vi "运维调试_总磷总氮.vi"() -> ()   [LabVIEW 2016, in "斯坦道总磷总氮V2.lvlib"]
uses:
  <vilib>/Utility/miscctls.llb/LVPointTypeDef.ctl
  <vilib>/Plasmionique/MB Master/MB_Master/MB_Master.lvclass
  <vilib>/ptbypt/NI_PtbyPt.lvlib
panel:
  in  "流程写入":bool
  in  "修改系列号":bool
  out "权限等级":string
  out "总步数":i32
  out "滑动杆":u8(slide) caption="测试进度" scale=0.0..100.0
  in  "关闭心跳包":bool
  in  "仪器校准":bool
  in  "参数查询":bool
  out "简易步骤名称":string
  in  "温度曲线":bool
  in  "启动参数设置":bool
  out "固件版本号":string
  in  "定时设置":cluster{"启动":bool, "控制命令":T1, "测量参数":T2}(xcontrol)
  out "模块版本号":string
  out "注射器温度":sgl
  out "消解温度":sgl
  out "ADC":sgl
  out "F3":sgl format="%#.6f"
  out "F2":sgl format="%#.6f"
  out "F1":sgl format="%#.6f"
  out "F0":sgl format="%#.6f"
  out "运行状态":T3 {"数据时间:" format="%<%y/%m/%d %H:%M:%S>T"; "仪器时间:" format="%<%y/%m/%d %H:%M:%S>T"}
  in  "单选按钮":T4(radio)=enum."总氮"
  in  "布尔":bool
  out "字符串 2":string
  in  "数组":string[](array[string])
  in  "返回":bool
  in  "参数设置":bool
  out "集成报警信息":string
  in  "停止":bool
  in  "手动启动":bool
  in  "调试":bool
  out "多列列表框":i32(listbox)
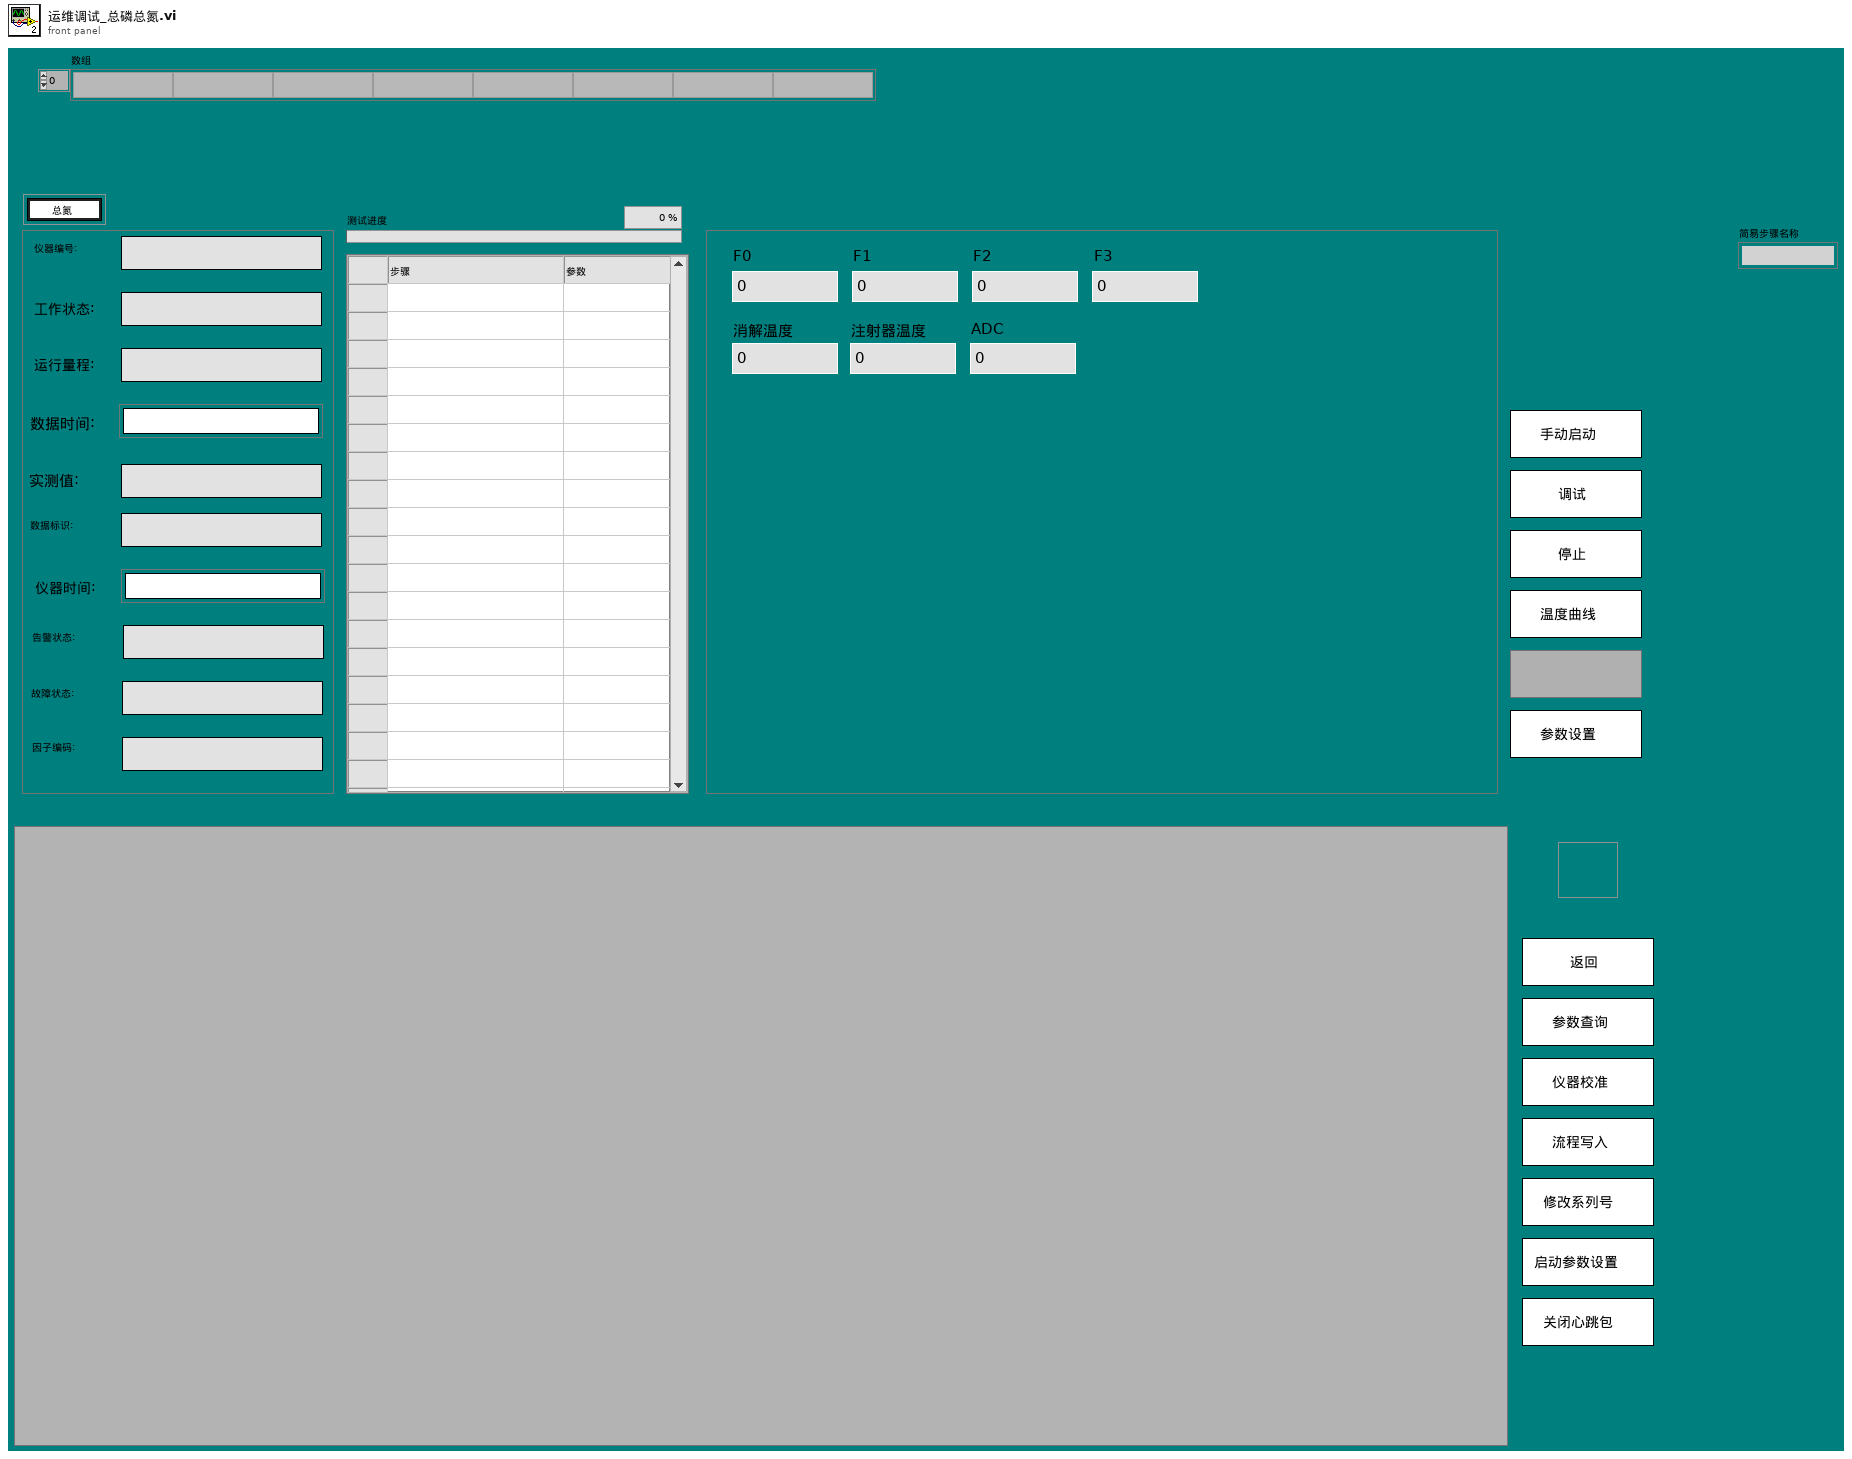
[diagram p1: front panel]
types:
  T1 = typedef "定时设置.xctl/国标控制命令.ctl" = enum16{"启动测量", "标样核查", "零点核查", "跨度核查", "空白测试", "平行样测试", "加标回收", "空白校准", "标样校准", "初始化（清洗）", "停止测试", "仪器重启", "校时", "模式设置", "测量间隔设置"}
  T2 = typedef "定时设置.xctl/测量参数.ctl" = u16
  T3 = cluster{"仪器编号:":string, "工作状态:":string, "运行量程: ":string, "数据时间:":timestamp, "实测值:":string, "数据标识: ":string, "仪器时间:":timestamp, "告警状态: ":string, "故障状态:  ":string, "因子编码:":string}
  T4 = enum32{"COD", "氨氮", "总氮", "总磷", "磷酸盐", "硝氮", "亚硝氮", "硅酸盐", "硫化物"}
  T5 = cluster{"Major":u16, "Minor":u16, "Fix":u16, "Build":u16}
  T6 = typedef "LVPointTypeDef.ctl" = cluster{"Horizontal":i16, "Vertical":i16}
  T7 = cluster{"系统时间":timestamp, "工作状态":u16, "测量模式":enum16{"待机", "连续模式", "周期模式", "定点模式", "受控模式", "手动模式"}, "告警代码":u16, "故障代码":u16, "日志代码":u16, "软件版本":u16, "F0":sgl, "F1":sgl, "F2":sgl, "F3":sgl, "T":sgl, "H":sgl, "id":u16, "flowid":u16, "量程":u16, "总磷控温温度1":sgl, "营养盐控温温度2":sgl, "ADC":sgl}
  T8 = cluster{"因子编码":u32, "单位":u16, "标样参考值":sgl, "水样数据时间":timestamp, "水样实测值":sgl, "水样数据标识":string, "标样数据时间":timestamp, "标样实测值":sgl, "标样数据标识":string, "空白数据时间":timestamp, "空白实测值":sgl, "空白数据标识":string, "零点核查数据时间":timestamp, "零点核查实测值":sgl, "零点核查数据标识":string, "跨度核查数据时间":timestamp, "跨度核查实测值":sgl, "跨度核查数据标识":string, "加标回收数据时间":timestamp, "加标回收实测值":sgl, "加标回收数据标识":string, "平行样数据时间":timestamp, "平行样实测值":sgl, "平行样数据标识":string, "F0":sgl, "F1":sgl, "F2":sgl, "F3":sgl, "F4":sgl, "F5":sgl, "F6":sgl, "F7":sgl, "温度":sgl, "湿度":sgl, "X值":sgl, "fidrange":u16}[]
  T9 = cluster{"因子编码":u32, "单位":u16, "标样参考值":sgl, "水样数据时间":timestamp, "水样实测值":sgl, "水样数据标识":string, "标样数据时间":timestamp, "标样实测值":sgl, "标样数据标识":string, "空白数据时间":timestamp, "空白实测值":sgl, "空白数据标识":string, "零点核查数据时间":timestamp, "零点核查实测值":sgl, "零点核查数据标识":string, "跨度核查数据时间":timestamp, "跨度核查实测值":sgl, "跨度核查数据标识":string, "加标回收数据时间":timestamp, "加标回收实测值":sgl, "加标回收数据标识":string, "平行样数据时间":timestamp, "平行样实测值":sgl, "平行样数据标识":string, "F0":sgl, "F1":sgl, "F2":sgl, "F3":sgl, "F4":sgl, "F5":sgl, "F6":sgl, "F7":sgl, "温度":sgl, "湿度":sgl, "X值":sgl, "fidrange":u16}
  T10 = cluster{"时间标识":timestamp, "设备":string, "日志信息":string, "备注":string}
  T11 = cluster{"参数":string, "报警内容":string, "报警分析":string}
  T12 = enum32{"Bad", "Idle", "Run top level", "Running"}
  T13 = enum16{"空闲", "水样测试", "标样核查", "零点核查", "跨度核查", "空白测试", "平行样测试", "加标回收", "空白校准", "标样校准", "初始化（清洗）"}
  T14 = cluster{"站号":u16, "量程切换":enum32{"H", "L", "AUTO"}, "控制命令":enum16{"启动测量", "标样核查", "零点核查", "跨度核查", "空白测试", "平行样测试", "加标回收", "空白校准", "标样校准", "初始化（清洗）", "停止测试", "仪器重启", "校时", "模式设置", "测量间隔设置"}, "模式设置":enum16{"待机", "连续模式", "周期模式", "定点模式", "受控模式", "手动模式"}, "测量间隔":u16}
  T15 = cluster{"时间标识":timestamp, "设备":string, "日志信息":string, "流程参数":string}
  T16 = typedef "LVRowAndColumnUnsignedTypeDef.ctl" = cluster{"Row":u32, "Column":u32}
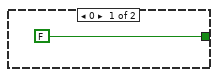
[diagram p3: hidden frame]
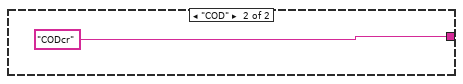
[diagram p4: hidden frame]
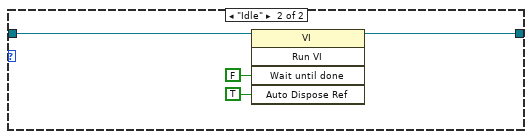
[diagram p7: hidden frame]
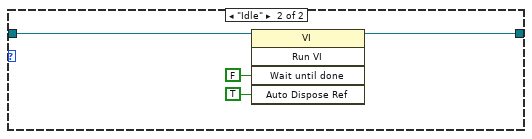
[diagram p8: hidden frame]
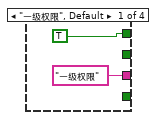
[diagram p14: hidden frame]
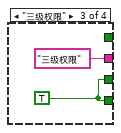
[diagram p15: hidden frame]
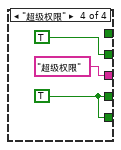
[diagram p16: hidden frame]
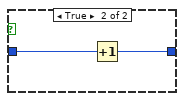
[diagram p18: hidden frame]
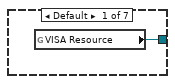
[diagram p20: hidden frame]
diagram:
  n1 = flat-sequence {
    tunnel: [w28] -> w17
    tunnel: [w29] -> w16
    tunnel: w17 -> [w40]
    tunnel: [w40] -> w2
    tunnel: w16 -> [_]
    tunnel: w2 -> [w63]
    tunnel: [w111] -> w18
    tunnel: [errorcluster {"status"=FALSE, "code"=0, "source"=""} ("错误输入（无错误）")] -> w7
    tunnel: [errorcluster {"status"=FALSE, "code"=0, "source"=""} ("错误输入（无错误）")] -> w6
    tunnel: [w108] -> w4
    tunnel: [errorcluster {"status"=FALSE, "code"=0, "source"=""} ("error out")] -> w1
    tunnel: [errorcluster {"status"=FALSE, "code"=0, "source"=""} ("错误输入（无错误）")] -> w3
    frame #0 {
      n2 = control-ref of="本VI"() -> (w30:refnum<vi>)
      n3 = control-ref of="本VI"() -> (w39:refnum<vi>)
      n4 = call "配置读取.vi"() -> ("error out"=w29:errorcluster)  [unwired: 11 in]
      n5 = property class="VI"(reference=w30) -> ("Library"=w31:refnum<vi>)  [unwired: 1 in, 2 out]
      n6 = property class="VI"(reference=w39) -> ("Library.Version"=w38:T5)  [unwired: 1 in, 2 out]
      n7 = property class="Library"(reference=w31) -> ("LocalName"=w28:string)  [unwired: 1 in, 2 out]
      n8 = Unbundle By Name(w38) -> ("Major"=w36:u16, "Minor"=w35:u16, "Fix"=w34:u16, "Build"=w33:u16)
      n9 = Search/Split String(string=w28, search string/char (-)="." ("搜索字符串/字符(-)")) -> (substring before match=w26:string)  [unwired: 1 in, 2 out]
      n10 = property on="定时设置" class="定时设置 (严格)"("调用模块名称写入"=w26) -> ()  [unwired: 2 in, 2 out]
      n11 = Format Into String(format string="模块版本号：%d.%d.%d.%d" ("格式字符串"), w36, w35, w34, w33) -> (resulting string=→"模块版本号":string)  [unwired: 2 in, 1 out]
    }
    frame #1 {
      n12 = global read "总磷总氮断电保存全局变量.vi" "IP"() -> (w44:string)
      n13 = global read "总磷总氮断电保存全局变量.vi" "VISA Resource"() -> (w41:refnum<visa-resource-name>)
      n14 = Empty String/Path?(string/path=w44) -> (empty?=w43:bool)
      n15 = Empty String/Path?(string/path=w41) -> (empty?=w42:bool)
      n16 = case shown="真" w43 {
        tunnel: w40 -> [_ w55]
        frame False {
        }
        frame True {
          n17 = case shown="\"斯坦道CODcrV2.lvlib\"" w55 {
            tunnel: [w56 "192.168.1.203" ("IP") "192.168.1.202" ("IP") "192.168.1.202" ("IP") "192.168.1.203" ("IP") "192.168.1.204" ("IP") "192.168.1.205" ("IP")] -> w54
            frame Default {
              n18 = global read "总磷总氮断电保存全局变量.vi" "IP"() -> (w56:string)
            }
            frame "斯坦道总磷总氮V2.lvlib" {
            }
            frame "斯坦道氨氮V2.lvlib" {
            }
            frame "斯坦道氨氮总磷V2.lvlib" {
            }
            frame "斯坦道总磷V2.lvlib" {
            }
            frame "斯坦道总氮V2.lvlib" {
            }
            frame "斯坦道CODcrV2.lvlib" {
            }
          }
          n19 = global write "总磷总氮断电保存全局变量.vi" "IP"(w54) -> ()
        }
      }
      n20 = case shown="真" w42 {
        tunnel: w40 -> [_ w46]
        frame False {
        }
        frame True {
          n21 = case shown="\"斯坦道总磷V2.lvlib\"" w46 {
            tunnel: [w47 "COM5" ("IP") "COM7" ("IP") "COM7" ("IP") "COM5" ("IP") "COM10" ("IP") "COM9" ("IP")] -> w45
            frame Default {
              n22 = global read "总磷总氮断电保存全局变量.vi" "VISA Resource"() -> (w47:refnum<visa-resource-name>)
            }
            frame "斯坦道总磷总氮V2.lvlib" {
            }
            frame "斯坦道氨氮V2.lvlib" {
            }
            frame "斯坦道氨氮总磷V2.lvlib" {
            }
            frame "斯坦道总磷V2.lvlib" {
            }
            frame "斯坦道总氮V2.lvlib" {
            }
            frame "斯坦道CODcrV2.lvlib" {
            }
          }
          n23 = global write "总磷总氮断电保存全局变量.vi" "VISA Resource"(w45) -> ()
        }
      }
    }
    frame #2 {
      n24 = global read "总磷总氮断电保存全局变量.vi" "启动队列名称"() -> (w65:cluster{"String":string, "Value":u16}[])
      n25 = Empty Array?(array=w65) -> (empty?=w64:bool)
      n26 = case shown="真" w64 {
        tunnel: w63 -> [_ w66]
        frame False {
        }
        frame True {
          n27 = case shown="\"斯坦道总氮V2.lvlib\"" w66 {
            frame Default {
            }
            frame "斯坦道总磷总氮V2.lvlib" {
              n28 = global write "总磷总氮断电保存全局变量.vi" "启动队列名称"(cluster{"String":string, "Value":u16}[] [{"String"="总氮", "Value"=2}, {"String"="总磷", "Value"=1}] ("启动队列名称")) -> ()
            }
            frame "斯坦道氨氮V2.lvlib" {
              n29 = global write "总磷总氮断电保存全局变量.vi" "启动队列名称"(cluster{"String":string, "Value":u16}[] [{"String"="氨氮", "Value"=3}] ("启动队列名称")) -> ()
            }
            frame "斯坦道氨氮总磷V2.lvlib" {
              n30 = global write "总磷总氮断电保存全局变量.vi" "启动队列名称"(cluster{"String":string, "Value":u16}[] [{"String"="氨氮", "Value"=3}, {"String"="总磷", "Value"=1}] ("启动队列名称")) -> ()
            }
            frame "斯坦道总磷V2.lvlib" {
              n31 = global write "总磷总氮断电保存全局变量.vi" "启动队列名称"(cluster{"String":string, "Value":u16}[] [{"String"="总磷", "Value"=1}] ("启动队列名称")) -> ()
            }
            frame "斯坦道总氮V2.lvlib" {
              n32 = global write "总磷总氮断电保存全局变量.vi" "启动队列名称"(cluster{"String":string, "Value":u16}[] [{"String"="总氮", "Value"=2}] ("启动队列名称")) -> ()
            }
            frame "斯坦道CODcrV2.lvlib" {
              n33 = global write "总磷总氮断电保存全局变量.vi" "启动队列名称"(cluster{"String":string, "Value":u16}[] [{"String"="CODcr", "Value"=22}] ("启动队列名称")) -> ()
            }
          }
        }
      }
    }
    frame #3 {
      # "初始化"
      n34 = global read "总磷总氮断电保存全局变量.vi" "流程路径"() -> (w76:path)
      n35 = global read "总磷总氮断电保存全局变量.vi" "启动队列名称"() -> (w73:cluster{"String":string, "Value":u16}[])
      n36 = call <vilib>:"Check if File or Folder Exists.vi"("path"=w76) -> ("file or folder exists?"=w80:bool)  [unwired: 8 in, 2 out]
      n37 = for {
        tunnel: w73 -> [w84] mode=indexing
        shift-right: [w83] -> w74
        shift-left: "" -> [w81]
        n38 = Unbundle By Name(w84) -> ("String"=w82:string)
        n39 = Concatenate Strings(w81, w82) -> (w83:string)
      }
      n40 = Empty String/Path?(string/path=w76) -> (empty?=w77:bool)
      n41 = Not(x=w80) -> (.not. x?=w79:bool)
      n42 = Or(x=w77, y=w79) -> (x .or. y?=w78:bool)
      n43 = case shown="真" w78 {
        frame False {
        }
        frame True {
          n44 = global read "总磷总氮断电保存全局变量.vi" "启动队列名称"() -> (w86:cluster{"String":string, "Value":u16}[])
          n45 = for {
            tunnel: w86 -> [w89] mode=indexing
            tunnel: [w88] -> w85 mode=indexing
            n46 = Unbundle By Name(w89) -> ("String"=w88:string)
          }
          n47 = call "获取默认流程路径.vi"("参数"=w85) -> ("路径"=w87:path)  [unwired: 10 in]
          n48 = global write "总磷总氮断电保存全局变量.vi" "流程路径"(w87) -> ()
        }
      }
      n49 = global write "VAR总磷总氮全局变量.vi" "模块名称"(w74) -> ()
    }
    frame #4 {
      n50 = vi-ref "总磷总氮测量数据储存.vi"() -> (w98:refnum<vi>)
      n51 = vi-ref "总磷总氮通讯.vi"() -> (w90:refnum<vi>)
      n52 = property class="VI"(reference=w98) -> ("Name"=w105:string)  [unwired: 1 in, 2 out]
      n53 = property class="VI"(reference=w90) -> ("Name"=w91:string)  [unwired: 1 in, 2 out]
      n54 = Open VI Reference(type specifier VI Refnum (for type only)=refnum<vi> refnum, vi path=w105, options=128 ("选项")) -> (vi reference=w103:refnum<vi>, error out=w101:errorcluster)  [unwired: 3 in]
      n55 = Open VI Reference(type specifier VI Refnum (for type only)=refnum<vi> refnum, vi path=w91, options=128 ("选项")) -> (vi reference=w93:refnum<vi>, error out=w95:errorcluster)  [unwired: 3 in]
      n56 = call-by-ref "开始异步调用"(reference=w103, error in=w101) -> (reference out=w99:refnum<vi>, error out=w100:errorcluster)  [unwired: 12 in]
      n57 = call-by-ref "开始异步调用"(reference=w93, error in=w95) -> (reference out=w97:refnum<vi>, error out=w96:errorcluster)  [unwired: 12 in]
      n58 = Close Reference(reference=w99, error in (no error)=w100) -> ()  [unwired: 1 out]
      n59 = Close Reference(reference=w97, error in (no error)=w96) -> ()  [unwired: 1 out]
    }
    frame #5 {
      n60 = call "配置文件路径.vi"() -> ("appended path"=w108:path)  [unwired: 11 in]
      n61 = call "设置模块队列名.vi"() -> ("Msg"=w111:string)  [unwired: 5 in]
    }
  }
  n62 = flat-sequence {
    frame #0 {
      n63 = property on="窗格" class="Pane"("Origin"=T6 {"Horizontal"=0, "Vertical"=0} ("原点")) -> ()  [unwired: 2 in, 2 out]
    }
  }
  n64 = while {
    shift-right: [w116] -> _
    shift-left: _ -> [w114]
    stop <- FALSE stop-if-true
    n65 = global read "VAR总磷总氮全局变量.vi" "状态告警区"() -> (w138:T7)
    n66 = global read "VAR总磷总氮全局变量.vi" "通讯状态"() -> (w149:bool)
    n67 = global write "VAR总磷总氮全局变量.vi" "最近一次工作状态"(w114) -> ()
    n68 = global read "VAR总磷总氮全局变量.vi" "状态告警区"() -> (w147:T7)
    n69 = Unbundle By Name(w138) -> ("id"=w137:u16, "工作状态"=w132:u16)
    n70 = case shown="真" w149 {
      tunnel: ["通讯异常" ("集成报警信息") w243] -> w148
      frame False {
      }
      frame True {
        n71 = global read "VAR总磷总氮全局变量.vi" "状态告警区"() -> (w249:T7)
        n72 = Unbundle By Name(w249) -> ("工作状态"=w248:u16)
        n73 = feedback #1(0) -> (w246:i32)
        n74 = case shown="0" w248 {
          tunnel: w246 -> [_ w251]
          tunnel: [_ w250] -> w244
          frame 0 {
          }
          frame Default {
            n75 = Increment(x=w251) -> (x+1=w250:i32)
          }
        }
        n76 = feedback-in #1(w244) -> ()
        n77 = global read "VAR总磷总氮全局变量.vi" "测量状态"() -> (w242:string)
        n78 = Format Into String(format string="工作计时: %d 秒" ("格式字符串"), initial string=w242, w244) -> (resulting string=w243:string)  [unwired: 1 in, 1 out]
      }
    }
    "集成报警信息" <- w148
    n79 = Unbundle By Name(w147) -> ("flowid"=w113:u16, "系统时间"=w143:timestamp, "工作状态"=w142:u16, "告警代码"=w136:u16, "故障代码"=w134:u16, "量程"=w141:u16)
    n80 = case shown="\"氨氮\"" "单选按钮" {
      tunnel: [22 3 2 1 4 5 6 7 8] -> w117
      frame "COD", Default {
      }
      frame "氨氮" {
      }
      frame "总氮" {
      }
      frame "总磷" {
      }
      frame "磷酸盐" {
      }
      frame "硝氮" {
      }
      frame "亚硝氮" {
      }
      frame "硅酸盐" {
      }
      frame "硫化物" {
      }
    }
    n81 = case shown="1, 默认" w132 {
      tunnel: w137 -> [_ w194]
      frame 0 {
      }
      frame 1, Default {
        n82 = case shown="3, 92" w194 {
          frame 0, Default {
          }
          frame 1, 131 {
            n83 = local write "单选按钮"(T4."总磷" ("单选按钮")) -> ()
          }
          frame 2, 76 {
            n84 = local write "单选按钮"(T4."总氮" ("单选按钮")) -> ()
          }
          frame 22 {
            n85 = local write "单选按钮"(T4."COD" ("单选按钮")) -> ()
          }
          frame 3, 92 {
            n86 = local write "单选按钮"(T4."氨氮" ("单选按钮")) -> ()
          }
          frame 4 {
            n87 = local write "单选按钮"(T4."磷酸盐" ("单选按钮")) -> ()
          }
          frame 5 {
            n88 = local write "单选按钮"(T4."硝氮" ("单选按钮")) -> ()
          }
          frame 6 {
            n89 = local write "单选按钮"(T4."亚硝氮" ("单选按钮")) -> ()
          }
          frame 7 {
            n90 = local write "单选按钮"(T4."硅酸盐" ("单选按钮")) -> ()
          }
          frame 8 {
            n91 = local write "单选按钮"(T4."硫化物" ("单选按钮")) -> ()
          }
        }
      }
    }
    n92 = case shown="255" w142 {
      selector: w142 -> [w208 _ w214 w218 w221 w223 w225 w227 w229 w231 w233 w235 w237 w240]
      tunnel: [w209 "空闲" ("工作状态") "水样测量" ("工作状态") w217 "零点核查" ("工作状态") "跨度核查" ("工作状态") "空白测试" ("工作状态") "平行样测试" ("工作状态") "加标回收" ("工作状态") "空白校准" ("工作状态") "标样校准" ("工作状态") "初始化" ("工作状态") "单步调试" ("工作状态") w239] -> w115
      tunnel: [w207 w212 w214 w218 w221 w223 w225 w227 w229 w231 w233 w235 w237 w240] -> w116
      tunnel: w114 -> [w207 w212 _ _ _ _ _ _ _ _ _ _ _ _]
      tunnel: w113 -> [_ _ _ w216 _ _ _ _ _ _ _ _ _ _]
      frame Default {
        n93 = Format Into String(format string="%d" ("格式字符串"), initial string="未知" ("工作状态"), w208) -> (resulting string=w209:string)  [unwired: 1 in, 1 out]
      }
      frame 0 {
      }
      frame 1 {
      }
      frame 2 {
        n94 = case shown="5" w216 {
          tunnel: ["标样核查" ("工作状态") "快捷测试" ("工作状态")] -> w217
          frame 0, Default {
          }
          frame 5 {
          }
        }
      }
      frame 3 {
      }
      frame 4 {
      }
      frame 5 {
      }
      frame 6 {
      }
      frame 7 {
      }
      frame 8 {
      }
      frame 9 {
      }
      frame 10 {
      }
      frame 254 {
      }
      frame 255 {
        n95 = local read "简易步骤名称"() -> (w239:string)
      }
    }
    n96 = case shown="1" w141 {
      tunnel: ["" ("字符串") "低量程 " ("字符串") "高量程 " ("字符串")] -> w140
      frame Default {
      }
      frame 0 {
      }
      frame 1 {
      }
    }
    n97 = Wait (ms)(milliseconds to wait=u32 1000 ("等待时间（毫秒）")) -> ()  [unwired: 1 out]
    n98 = call "id参数转换.vi"("id"=w117) -> ("数组资源索引"=w118:i32)  [unwired: 9 in, 1 out]
    n99 = global read "VAR总磷总氮全局变量.vi" "测量数据区数组"() -> (w121:T8)
    n100 = Index Array(array=w121, index=w118) -> (element=w120:T9)
    n101 = case shown="0, 默认" w114 {
      tunnel: [w163 w169 w173 w177 w181 w185 w189 w193] -> w131
      tunnel: [w161 w168 w172 w176 w179 w184 w188 w192] -> w126
      tunnel: [w164 w167 w171 w175 w178 w183 w187 w191] -> w124
      tunnel: w120 -> [_ w166 w170 w174 w180 w182 w186 w190]
      frame 0, Default {
        n102 = local read "运行状态"() -> (w165:T3)
        n103 = Unbundle By Name(w165) -> ("数据时间:"=w163:timestamp, "实测值:"=w162:string, "数据标识:"=w164:string)
        n104 = Fract/Exp String To Number(string=w162) -> (number=w161:dbl)  [unwired: 3 in, 1 out]
      }
      frame 1 {
        n105 = Unbundle By Name(w166) -> ("水样数据时间"=w169:timestamp, "水样实测值"=w168:sgl, "水样数据标识"=w167:string)
      }
      frame 2, 9 {
        n106 = Unbundle By Name(w170) -> ("标样数据时间"=w173:timestamp, "标样实测值"=w172:sgl, "标样数据标识"=w171:string)
      }
      frame 3 {
        n107 = Unbundle By Name(w174) -> ("零点核查数据时间"=w177:timestamp, "零点核查实测值"=w176:sgl, "零点核查数据标识"=w175:string)
      }
      frame 4 {
        n108 = Unbundle By Name(w180) -> ("跨度核查数据时间"=w181:timestamp, "跨度核查实测值"=w179:sgl, "跨度核查数据标识"=w178:string)
      }
      frame 7 {
        n109 = Unbundle By Name(w182) -> ("加标回收数据时间"=w185:timestamp, "加标回收实测值"=w184:sgl, "加标回收数据标识"=w183:string)
      }
      frame 5, 8 {
        n110 = Unbundle By Name(w186) -> ("空白数据时间"=w189:timestamp, "空白实测值"=w188:sgl, "空白数据标识"=w187:string)
      }
      frame 6 {
        n111 = Unbundle By Name(w190) -> ("平行样数据时间"=w193:timestamp, "平行样实测值"=w192:sgl, "平行样数据标识"=w191:string)
      }
    }
    n112 = Unbundle By Name(w120) -> ("因子编码"=w122:u32)
    n113 = global write "VAR总磷总氮全局变量.vi" "工作状态:"(w115) -> ()
    n114 = Format Into String(format string="w%05d" ("格式字符串"), w122) -> (resulting string=w139:string)  [unwired: 2 in, 1 out]
    n115 = Number To Fractional String(number=w126, precision (6)=i16 4 ("精度(6)")) -> (F-format string=w128:string)  [unwired: 2 in]
    n116 = call "告警码字段定义.vi"("告警代码"=w136) -> ("字符串"=w135:string)  [unwired: 8 in, 2 out]
    n117 = call "故障码字段定义.vi"("故障代码"=w134) -> ("字符串"=w133:string)  [unwired: 10 in]
    n118 = Concatenate Strings(w128, " " ("字符串"), "mg/L" ("字符串")) -> (w125:string)
    n119 = global read "VAR总磷总氮全局变量.vi" "序列号"() -> (w144:string)
    n120 = Bundle By Name(cluster=T3 {"仪器编号:"="", "工作状态:"="", "运行量程: "="", "数据时间:"=timestamp(0 s since 1904-01-01), "实测值:"="", "数据标识: "="", "仪器时间:"=timestamp(0 s since 1904-01-01), "告警状态: "="", "故障状态:  "="", "因子编码:"=""} ("运行状态"), "仪器编号:"=w144, "仪器时间:"=w143, "工作状态:"=w115, "告警状态:"=w135, "故障状态:"=w133, "运行量程:"=w140, "数据时间:"=w131, "实测值:"=w125, "数据标识:"=w124, "因子编码:"=w139) -> (→"运行状态":T3)
  }
  n121 = call "Create balloon 队列.vi"() -> ("队列输出"=w22:refnum<queue>)  [unwired: 11 in]
  n122 = while {
    shift-right: [w255] -> _
    shift-left: _ -> [w254]
    stop <- FALSE stop-if-true
    n123 = global read "VAR总磷总氮全局变量.vi" "状态告警区"() -> (w257:T7)
    n124 = Unbundle By Name(w257) -> ("工作状态"=w256:u16, "总磷控温温度1"=w253:sgl, "营养盐控温温度2"=w252:sgl)
    n125 = case shown="默认" w256 {
      tunnel: [TRUE _] -> w255
      tunnel: w254 -> [w266 _]
      tunnel: w253 -> [w264 _]
      tunnel: w252 -> [w262 _]
      frame Default {
        n126 = case shown="真" w266 {
          tunnel: [_ w269] -> w265
          tunnel: [_ w268] -> w263
          frame False {
          }
          frame True {
            n127 = global read "VAR总磷总氮全局变量.vi" "波形图-消解温度"() -> (w269:dbl[])
            n128 = global read "VAR总磷总氮全局变量.vi" "波形图-注射器温度"() -> (w268:dbl[])
          }
        }
        n129 = Insert Into Array(array=w265, new element=w264) -> (w261:dbl[])  [unwired: 1 in]
        n130 = Insert Into Array(array=w263, new element=w262) -> (w260:dbl[])  [unwired: 1 in]
        n131 = global write "VAR总磷总氮全局变量.vi" "波形图-消解温度"(w261) -> ()
        n132 = global write "VAR总磷总氮全局变量.vi" "波形图-注射器温度"(w260) -> ()
      }
      frame 0, 254, 255 {
      }
    }
    n133 = Wait (ms)(milliseconds to wait=u32 1000 ("等待时间（毫秒）")) -> ()  [unwired: 1 out]
  }
  n134 = while {
    shift-right: [w280] -> _
    shift-left: u32 0 ("y") -> [w282]
    stop <- FALSE stop-if-true
    # "密码权限"
    n135 = global read "VAR总磷总氮全局变量.vi" "权限等级"() -> (w277:enum16{"一级权限", "二级权限", "三级权限", "超级权限"})
    n136 = case shown="\"二级权限\"" w277 {
      tunnel: [_ TRUE w289 w292] -> w270
      tunnel: [_ _ w289 w292] -> w271
      tunnel: [_ _ _ TRUE] -> w276
      tunnel: [TRUE _ _ _] -> w274
      tunnel: ["一级权限" "二级权限" "三级权限" "超级权限"] -> w272
      frame "一级权限", Default {
      }
      frame "二级权限" {
      }
      frame "三级权限" {
        w289 = TRUE
      }
      frame "超级权限" {
        w292 = TRUE
      }
    }
    "权限等级" <- w272
    n137 = case shown="假" "布尔" {
      tunnel: w282 -> [_ w295]
      tunnel: [_ w294] -> w280
      frame False {
      }
      frame True {
        n138 = Increment(x=w295) -> (x+1=w294:u32)
      }
    }
    n139 = Wait (ms)(milliseconds to wait=u32 1000 ("等待时间（毫秒）")) -> ()  [unwired: 1 out]
    n140 = Not(x=w274) -> (.not. x?=w273:bool)
    n141 = property on="关闭心跳包" class="Bool (严格)"("Visible"=w276) -> ()  [unwired: 2 in, 2 out]
    n142 = property on="流程写入" class="Bool"("Visible"=w270) -> ()  [unwired: 2 in, 2 out]
    n143 = property on="修改系列号" class="Bool"("Visible"=w271) -> ()  [unwired: 2 in, 2 out]
    n144 = property on="启动参数设置" class="Bool"("Visible"=w271) -> ()  [unwired: 2 in, 2 out]
    n145 = Greater Or Equal?(x=w280, y=u32 3600) -> (x >= y?=w278:bool)
    n146 = property on="布尔" class="Bool (严格)"("Value"=w273) -> ()  [unwired: 2 in, 2 out]
    n147 = case shown="真" w278 {
      frame False {
      }
      frame True {
        n148 = global write "VAR总磷总氮全局变量.vi" "权限等级"(enum16{"一级权限", "二级权限", "三级权限", "超级权限"}."一级权限" ("权限等级")) -> ()
      }
    }
  }
  n149 = while {
    shift-right: [w300] -> _
    shift-left: 0 -> [w301]
    stop <- FALSE stop-if-true
    n150 = global read "VAR总磷总氮全局变量.vi" "心跳包打开状态"() -> (w296:bool)
    n151 = case shown="假" w296 {
      tunnel: w301 -> [w305 _]
      tunnel: [w304 _] -> w300
      frame False {
        n152 = Increment(x=w305) -> (x+1=w304:i32)
      }
      frame True {
      }
    }
    n153 = Wait (ms)(milliseconds to wait=u32 1000 ("等待时间（毫秒）")) -> ()  [unwired: 1 out]
    n154 = Greater Or Equal?(x=w300, y=3600) -> (x >= y?=w298:bool)
    n155 = case shown="真" w298 {
      frame False {
      }
      frame True {
        w303 = FALSE ("关闭心跳包")
        n156 = local write "关闭心跳包"(w303) -> ()
        n157 = global write "VAR总磷总氮全局变量.vi" "升级固件关闭心跳包"(w303) -> ()
      }
    }
  }
  n158 = while {
    tunnel: w22 -> [w312]
    shift-right: [w308] -> _
    shift-left: _ -> [w309]
    stop <- FALSE stop-if-true
    n159 = global read "VAR总磷总氮全局变量.vi" "状态告警区"() -> (w306:T7)
    n160 = Unbundle By Name(w306) -> ("工作状态"=w307:u16, "id"=w314:u16, "日志代码"=w313:u16, "故障代码"=w311:u16, "告警代码"=w310:u16)
    n161 = case shown="1, 默认" w307 {
      tunnel: w314 -> [_ w329]
      tunnel: w313 -> [_ w328]
      tunnel: w312 -> [_ w325]
      tunnel: w311 -> [_ w324]
      tunnel: w310 -> [_ w323]
      tunnel: w309 -> [w317 w322]
      tunnel: [w317 w321] -> w308
      frame 0 {
      }
      frame 1, Default {
        n162 = Add(x=w324, y=w323) -> (x+y=w321:u16)
        n163 = call "id参数转换.vi"("id"=w329) -> ("table输出"=w326:string)  [unwired: 9 in, 1 out]
        n164 = Not Equal To 0?(x=w321) -> (x != 0?=w320:bool)
        n165 = Not Equal?(x=w321, y=w322) -> (x != y?=w319:bool)
        n166 = call "故障告警分析.vi"("告警代码"=w323, "故障代码"=w324, "运行步序"=w328, "参数"=w326) -> ("报警内容"=w327:T11)  [unwired: 6 in, 1 out]
        n167 = And(x=w320, y=w319) -> (x .and. y?=w318:bool)
        n168 = case shown="真" w318 {
          tunnel: w327 -> [_ w338]
          tunnel: w325 -> [_ w337]
          frame False {
          }
          frame True {
            n169 = Get Date/Time In Seconds() -> (seconds since 1Jan1904=w336:timestamp)
            n170 = Unbundle By Name(w338) -> ("参数"=w333:string, "报警内容"=w332:string, "报警分析"=w331:string)
            n171 = Bundle("报警内容"=w332, "报警分析"=w331) -> (w330:cluster{"报警内容":string, "报警分析":string})  [unwired: 1 in]
            n172 = Bundle By Name(cluster=T10 {"时间标识"=timestamp(0 s since 1904-01-01), "设备"="", "日志信息"="", "备注"=""} ("data in"), "时间标识"=w336, "设备"=w333, "日志信息"=w332, "备注"=w331) -> (w335:T10)
            n173 = call "总磷总氮报警信息.vi"("data in"=w335) -> ()  [unwired: 10 in, 1 out]
            n174 = call "balloon入队列.vi"("报警内容"=w330, "队列"=w337) -> ()  [unwired: 9 in, 1 out]
          }
        }
      }
    }
    n175 = Wait (ms)(milliseconds to wait=u32 100) -> ()  [unwired: 1 out]
  }
  n176 = flat-sequence {
    tunnel: w1 -> [_]
    frame #0 {
      n177 = call "taskqueue ref.vi"() -> ("队列输出"=w339:refnum<queue>)  [unwired: 10 in, 1 out]
      n178 = while {
        tunnel: w339 -> [w345]
        stop <- FALSE stop-if-true
        n179 = global read "VAR总磷总氮全局变量.vi" "状态告警区"() -> (w349:T7)
        n180 = Unbundle By Name(w349) -> ("工作状态"=w348:u16, "系统时间"=w340:timestamp)
        n181 = Unbundle By Name("定时设置") -> ("启动"=w343:bool, "控制命令"=w344:T1)
        n182 = case shown="1, 默认" w348 {
          tunnel: [FALSE TRUE] -> w346
          frame 0 {
          }
          frame 1, Default {
          }
        }
        n183 = call <vilib>:"Boolean Crossing PtByPt.vi"("direction"=enum16{"either", "false-true", "true-false"}."false-true", "input"=w343) -> ("crossing"=w341:bool)  [unwired: 1 in]
        n184 = case shown="真" w341 {
          tunnel: w345 -> [_ w353]
          tunnel: w344 -> [_ w352]
          frame False {
          }
          frame True {
            n185 = Enqueue Element(queue=w353, element=w352) -> ()  [unwired: 2 in, 3 out]
          }
        }
        n186 = Wait (ms)(milliseconds to wait=u32 500 ("等待时间（毫秒）")) -> ()  [unwired: 1 out]
        n187 = property on="定时设置" class="定时设置 (严格)"("仪器状态"=w346, "仪器时间写入"=w340) -> ()  [unwired: 2 in, 2 out]
      }
      n188 = call "task.vi"() -> ()  [unwired: 12 in]
    }
  }
  n189 = while {
    shift-right: [w359] -> _
    shift-left: _ -> [w361]
    tunnel: w4 -> [w358]
    stop <- FALSE stop-if-true
    n190 = Read from Text File(file (use dialog)=w358) -> (text=w359:string, error out=w356:errorcluster)  [unwired: 3 in, 2 out]
    n191 = Not Equal?(x=w361, y=w359) -> (x != y?=w360:bool)
    n192 = case shown="真" w360 {
      tunnel: [_ w363] -> _
      tunnel: w356 -> [_ _]
      frame False {
      }
      frame True {
        n193 = call "配置读取.vi"() -> ("error out"=w363:errorcluster)  [unwired: 11 in]
      }
    }
    n194 = Wait (ms)(milliseconds to wait=u32 1000 ("等待时间（毫秒）")) -> ()  [unwired: 1 out]
  }
  n195 = vi-ref "校准设置页.vi"() -> (w11:refnum<vi>)
  n196 = vi-ref "参数设置页.vi"() -> (w15:refnum<vi>)
  n197 = call "时间延迟"("error in (no error)"=w3) -> ("error out"=w25:errorcluster)  [unwired: 10 in]
  n198 = Obtain Notifier(name (unnamed)=w18, notification data type=FALSE) -> (notifier out=w19:refnum<notifier>)  [unwired: 2 in, 2 out]
  n199 = Obtain Queue(name (unnamed)=w18, element data type=cluster{"命令":string, "data":variant} {"命令"="", "data"=variant}) -> (queue out=w21:refnum<queue>)  [unwired: 3 in, 2 out]
  n200 = while {
    tunnel: w1 -> [_]
    stop <- FALSE stop-if-true
    n201 = flat-sequence {
      frame #0 {
        n202 = global read "总磷总氮断电保存全局变量.vi" "启动队列名称"() -> (w368:cluster{"String":string, "Value":u16}[])
        n203 = global read "总磷总氮断电保存全局变量.vi" "启动队列名称"() -> (w366:cluster{"String":string, "Value":u16}[])
        n204 = for {
          tunnel: w368 -> [w374] mode=indexing
          shift-right: [w373] -> w369
          shift-left: "" -> [w371]
          n205 = Unbundle By Name(w374) -> ("String"=w372:string)
          n206 = Concatenate Strings(w371, w372) -> (w373:string)
        }
        n207 = for {
          tunnel: w366 -> [w376] mode=indexing
          tunnel: [w375] -> w367 mode=indexing
          n208 = Unbundle By Name(w376) -> ("String"=w375:string)
        }
        n209 = property on="单选按钮" class="RadioBtnsControl (严格)"() -> ("Controls[]"=w365:refnum<vi>[])  [unwired: 2 in, 2 out]
        n210 = global write "VAR总磷总氮全局变量.vi" "模块名称"(w369) -> ()
        n211 = for {
          tunnel: w365 -> [w384] mode=indexing
          tunnel: w367 -> [w383]
          n212 = property class="Ctl"(reference=w384) -> (reference out=w382:refnum<vi>, "Label.Text"=w378:string)  [unwired: 1 in, 1 out]
          n213 = case shown="默认" w378 {
            selector: w378 -> [w385 _]
            tunnel: [w385 "CODcr"] -> w377
            frame Default {
            }
            frame "COD" {
            }
          }
          n214 = Search 1D Array(1D array=w383, element=w377) -> (index of element=w381:i32)  [unwired: 1 in]
          n215 = Not Equal?(x=w381, y=-1) -> (x != y?=w379:bool)
          n216 = property class="Ctl"(reference=w382, "Visible"=w379) -> ()  [unwired: 1 in, 2 out]
        }
      }
      frame #1 {
        n217 = Wait (ms)(milliseconds to wait=u32 5000 ("等待时间（毫秒）")) -> ()  [unwired: 1 out]
      }
    }
  }
  n218 = property class="VI"(reference=w11, error in=w6) -> (reference out=w9:refnum<vi>, "Exec.State"=w10:T12)  [unwired: 1 out]
  n219 = property class="VI"(reference=w15, error in=w7) -> (reference out=w13:refnum<vi>, "Exec.State"=w14:T12)  [unwired: 1 out]
  n220 = while {
    tunnel: w21 -> [w401]
    stop <- FALSE stop-if-true
    n221 = global read "总磷总氮断电保存全局变量.vi" "MB通信方式选择"() -> (w399:enum16{"串口", "TCP"})
    n222 = Get Queue Status(queue=w401) -> (queue out=w400:refnum<queue>, # elements in queue=w396:i32)  [unwired: 2 in, 6 out]
    n223 = global read "VAR总磷总氮全局变量.vi" "MB session in"() -> (w397:refnum<class "MB_Master.lvclass">)
    n224 = global read "VAR总磷总氮全局变量.vi" "升级固件关闭心跳包"() -> (w391:bool)
    n225 = Not(x="关闭心跳包") -> (.not. x?=w393:bool)
    n226 = Not(x=w391) -> (.not. x?=w390:bool)
    n227 = case shown="\"串口\", 默认" w399 {
      tunnel: [w404 w405] -> w398
      frame "串口", Default {
        n228 = global read "总磷总氮断电保存全局变量.vi" "VISA Resource"() -> (w404:refnum<visa-resource-name>)
      }
      frame "TCP" {
        n229 = global read "总磷总氮断电保存全局变量.vi" "IP"() -> (w405:string)
      }
    }
    "字符串 2" <- w398
    n230 = property class="MB_Master"(reference=w397) -> ("Properties:Session Valid"=w395:bool)  [unwired: 1 in, 2 out]
    n231 = Compound Arithmetic op=AND ("复合运算")(w395, w393, w390) -> (w392:bool)
    n232 = Equal To 0?(x=w396) -> (x = 0?=w388:bool)
    n233 = global write "VAR总磷总氮全局变量.vi" "心跳包打开状态"(w392) -> ()
    n234 = And(x=w392, y=w388) -> (x .and. y?=w389:bool)
    n235 = case shown="真" w389 {
      tunnel: w400 -> [_ w419]
      frame False {
      }
      frame True {
        n236 = global read "VAR总磷总氮全局变量.vi" "状态告警区"() -> (w411:T7)
        n237 = global read "总磷总氮断电保存全局变量.vi" "启动队列名称"() -> (w408:cluster{"String":string, "Value":u16}[])
        n238 = Unbundle By Name(w411) -> ("系统时间"=w418:timestamp, "工作状态"=w410:u16)
        n239 = for {
          tunnel: [w437] -> w409 mode=indexing
          tunnel: w408 -> [w438] mode=indexing
          n240 = Unbundle By Name(w438) -> ("Value"=w437:u16)
        }
        n241 = Get Date/Time In Seconds() -> (seconds since 1Jan1904=w417:timestamp)
        n242 = Subtract(x=w417, y=w418) -> (x-y=w416:dbl)
        n243 = Absolute Value(x=w416) -> (abs(x)=w415:dbl)
        n244 = for {
          tunnel: w410 -> [w423]
          shift-right: [w424] -> w412
          shift-left: w419 -> [w426]
          tunnel: w409 -> [w420] mode=indexing
          n245 = Equal?(x=w423, y=T13."空闲") -> (x = y?=w421:bool)
          n246 = Bundle By Name(cluster=cluster{"命令":string, "data":variant} {"命令"="", "data"=variant} ("元素"), "命令"="读状态告警区", "data"=w420) -> (w428:cluster{"命令":string, "data":variant})
          n247 = Enqueue Element(queue=w426, element=w428) -> (queue out=w425:refnum<queue>)  [unwired: 2 in, 2 out]
          n248 = case shown="真" w421 {
            tunnel: w425 -> [w430 w433]
            tunnel: w420 -> [_ w432]
            tunnel: [w430 w431] -> w424
            frame False {
            }
            frame True {
              n249 = Bundle By Name(cluster=cluster{"命令":string, "data":variant} {"命令"="", "data"=variant} ("元素"), "命令"="读测量数据区", "data"=w432) -> (w435:cluster{"命令":string, "data":variant})
              n250 = Enqueue Element(queue=w433, element=w435) -> (queue out=w431:refnum<queue>)  [unwired: 2 in, 2 out]
            }
          }
        }
        n251 = Greater Or Equal?(x=w415, y=120.0) -> (x >= y?=w413:bool)
        n252 = global read "VAR总磷总氮全局变量.vi" "通讯状态"() -> (w406:bool)
        n253 = And(x=w413, y=w406) -> (x .and. y?=w407:bool)
        n254 = case shown="假" w407 {
          tunnel: w412 -> [_ w446]
          tunnel: [w439 _] -> _
          frame False {
            n255 = global read "VAR总磷总氮全局变量.vi" "MB session in"() -> (w442:refnum<class "MB_Master.lvclass">)
            n256 = call "版本号读取.vi"("MB session in"=w442) -> ("error out"=w440:errorcluster, "固件版本号"=→"固件版本号":string, "MB session out"=w441:refnum<class "MB_Master.lvclass">)  [unwired: 8 in]
            n257 = call "序列号读取.vi"("Error in"=w440, "MB session in"=w441) -> ("error out"=w439:errorcluster, "序列号"=w444:string)  [unwired: 7 in, 1 out]
            n258 = global write "VAR总磷总氮全局变量.vi" "序列号"(w444) -> ()
          }
          frame True {
            n259 = call "总磷总氮启动命令.vi"("参数"=T14 {"站号"=3, "量程切换"=enum."AUTO", "控制命令"=enum."校时", "模式设置"=enum."待机", "测量间隔"=0}) -> ("启动命令"=w445:cluster{"命令":string, "data":variant})  [unwired: 10 in]
            n260 = Enqueue Element(queue=w446, element=w445) -> ()  [unwired: 2 in, 3 out]
          }
        }
      }
    }
    n261 = Wait (ms)(milliseconds to wait=u32 1000 ("等待时间（毫秒）")) -> ()  [unwired: 1 out]
  }
  n262 = while {
    tunnel: w25 -> [_]
    stop <- FALSE stop-if-true
    n263 = global read "VAR总磷总氮全局变量.vi" "状态告警区"() -> (w480:T7)
    n264 = global read "VAR总磷总氮全局变量.vi" "状态告警区"() -> (w478:T7)
    n265 = global read "VAR总磷总氮全局变量.vi" "状态告警区"() -> (w481:T7)
    n266 = global read "VAR总磷总氮全局变量.vi" "状态告警区"() -> (w482:T7)
    n267 = Unbundle By Name(w480) -> ("flowid"=w449:u16, "工作状态"=w470:u16, "id"=w471:u16)
    n268 = Unbundle By Name(w478) -> ("日志代码"=w477:u16)
    n269 = Unbundle By Name(w481) -> ("日志代码"=w452:u16)
    n270 = Unbundle By Name(w482) -> ("id"=w457:u16, "flowid"=w456:u16, "量程"=w455:u16, "工作状态"=w459:u16, "日志代码"=w454:u16, "F0"=→"F0":sgl, "F1"=→"F1":sgl, "F2"=→"F2":sgl, "F3"=→"F3":sgl, "ADC"=→"ADC":sgl, "总磷控温温度1"=→"消解温度":sgl, "营养盐控温温度2"=→"注射器温度":sgl)
    n271 = Not Equal To 0?(x=w470) -> (x != 0?=w468:bool)
    n272 = case shown="0" w470 {
      frame 0 {
        n273 = local write "数组"(string[] [] ("数组")) -> ()
      }
      frame 1, Default {
      }
    }
    n274 = feedback #2(w477) -> (w479:u16)
    n275 = feedback-in #2(w477) -> ()
    n276 = feedback-in #3(w452) -> ()
    n277 = feedback #3(w452) -> (w484:u16)
    n278 = property on="总步数" class="DigNum (严格)"() -> ("Value"=w453:i32)  [unwired: 2 in, 2 out]
    n279 = Subtract(x=w452, y=1) -> (x-y=→"多列列表框":i32)
    n280 = Not Equal?(x=w477, y=w479) -> (x != y?=w476:bool)
    n281 = Not Equal?(x=w452, y=w484) -> (x != y?=w483:bool)
    n282 = Divide(x=w452, y=w453) -> (x/y=w451:dbl)
    n283 = Bundle("id"=w457, "flowid"=w456, "量程"=w455) -> (w458:cluster{"id":u16, "flowid":u16, "量程":u16})  [unwired: 1 in]
    n284 = call <vilib>:"Boolean Crossing PtByPt.vi"("direction"=enum16{"either", "false-true", "true-false"}."false-true", "input"=w468) -> ("crossing"=w472:bool)  [unwired: 1 in]
    n285 = call <vilib>:"Boolean Crossing PtByPt.vi"("direction"=enum16{"either", "false-true", "true-false"}."true-false", "input"=w468) -> ("crossing"=w467:bool)  [unwired: 1 in]
    n286 = case shown="真" w476 {
      frame False {
      }
      frame True {
        n287 = property on="多列列表框" class="MCListbox (严格)"() -> ("ItemNames"=w556:string[][], "Value"=w552:i32)  [unwired: 2 in, 2 out]
        n288 = Index Array(array=w556, index (row)=w552) -> (element=w555:string[])  [unwired: 1 in]
        n289 = Index Array(array=w555) -> (element=w554:string)  [unwired: 1 in]
        n290 = call "过滤筛选流程.vi"("字符串"=w554) -> ("匹配后偏移量"=w553:i32)  [unwired: 10 in]
        n291 = case shown="默认" w553 {
          tunnel: w554 -> [w558 _]
          tunnel: w552 -> [w557 _]
          frame Default {
            n292 = case shown="默认" w558 {
              selector: w558 -> [w564 w571]
              tunnel: [w564 w571] -> w560
              tunnel: [string[] [] ("数组") w566] -> w559
              tunnel: w557 -> [_ w570]
              frame "读数" {
              }
              frame Default {
                n293 = Equal?(x=w570, y=1) -> (x = y?=w568:bool)
                n294 = Select(t=string[] [], s=w568, f="数组") -> (s? t:f=w566:string[])
              }
            }
            n295 = for {
              N: 1 -> [_]
              tunnel: w560 -> [w573]
              shift-right: [w572] -> w561
              shift-left: w559 -> [w574]
              n296 = Search 1D Array(1D array=w574, element=w573) -> (index of element=w577:i32)  [unwired: 1 in]
              n297 = Format Into String(format string="%s" ("格式字符串"), w573) -> (resulting string=w578:string)  [unwired: 2 in, 1 out]
              n298 = Equal?(x=w577, y=-1) -> (x = y?=w575:bool)
              n299 = case shown="真" w575 {
                tunnel: w578 -> [_ w588]
                tunnel: w574 -> [w580 w592]
                tunnel: w573 -> [_ w591]
                tunnel: [w580 w590] -> w572
                frame False {
                }
                frame True {
                  n300 = global read "VAR总磷总氮全局变量.vi" "状态告警区"() -> (w587:T7)
                  n301 = global read "VAR总磷总氮全局变量.vi" "状态告警区"() -> (w602:T7)
                  n302 = global read "VAR总磷总氮全局变量.vi" "状态告警区"() -> (w605:T7)
                  n303 = Insert Into Array(array=w592, new element=w591) -> (w590:string[])  [unwired: 1 in]
                  n304 = Unbundle By Name(w587) -> ("工作状态"=w586:u16, "flowid"=w581:u16)
                  n305 = Unbundle By Name(w602) -> ("F0"=w599:sgl, "F1"=w598:sgl, "F2"=w597:sgl, "F3"=w596:sgl, "id"=w595:u16, "flowid"=w594:u16, "量程"=w593:u16)
                  n306 = Unbundle By Name(w605) -> ("id"=w583:u16)
                  n307 = case shown="1" w586 {
                    selector: w586 -> [w607 _ _ _ _ _ _ _ _ _ _ _]
                    tunnel: [w606 "【水样测试】" ("字符串") w610 "【零点核查】" ("字符串") "【跨度核查】" ("字符串") "【空白测试】" ("字符串") "【平行样测试】" ("字符串") "【加标回收】" ("字符串") "【空白校准】" ("字符串") "【标样校准】" ("字符串") "【单步调试】" ("字符串") w621] -> w584
                    tunnel: w581 -> [_ _ w609 _ _ _ _ _ _ _ _ _]
                    frame 0, Default {
                      n308 = Number To Decimal String(number=w607) -> (decimal integer string=w606:string)  [unwired: 1 in]
                    }
                    frame 1 {
                    }
                    frame 2 {
                      n309 = case shown="默认" w609 {
                        tunnel: ["【标样核查】" ("字符串") "【快捷测试】" ("字符串")] -> w610
                        frame Default {
                        }
                        frame 5 {
                        }
                      }
                    }
                    frame 3 {
                    }
                    frame 4 {
                    }
                    frame 5 {
                    }
                    frame 6 {
                    }
                    frame 7 {
                    }
                    frame 8 {
                    }
                    frame 9 {
                    }
                    frame 254 {
                    }
                    frame 255 {
                      n310 = local read "简易步骤名称"() -> (w623:string)
                      n311 = Format Into String(format string="(%s)" ("格式字符串"), initial string="【简易流程】" ("工作状态"), w623) -> (resulting string=w621:string)  [unwired: 1 in, 1 out]
                    }
                  }
                  n312 = call "id参数转换.vi"("id"=w583) -> ("table输出"=w582:string)  [unwired: 9 in, 1 out]
                  n313 = Format Into String(format string="F0=%#f,F1=%#f,F2=%#f,F3=%#f,Flow=%d-%-d-%-d" ("格式字符串"), w599, w598, w597, w596, w595, w594, w593) -> (resulting string=w600:string)  [unwired: 2 in, 1 out]
                  n314 = Concatenate Strings(w584, w588) -> (w585:string)
                  n315 = Get Date/Time In Seconds() -> (seconds since 1Jan1904=w603:timestamp)
                  n316 = Bundle By Name(cluster=T15 {"时间标识"=timestamp(0 s since 1904-01-01), "设备"="", "日志信息"="", "流程参数"=""} ("data in"), "时间标识"=w603, "设备"=w582, "日志信息"=w585, "流程参数"=w600) -> (w604:T15)
                  n317 = call "总磷总氮操作日志.vi"("data in"=w604) -> ()  [unwired: 10 in, 1 out]
                }
              }
            }
            n318 = local write "数组"(w561) -> ()
          }
          frame -1 {
          }
        }
      }
    }
    n319 = case shown="真" w483 {
      tunnel: w452 -> [_ w656]
      frame False {
      }
      frame True {
        n320 = Subtract(x=w656, y=1) -> (x-y=w654:i32)
        n321 = Subtract(x=w654, y=5) -> (x-y=w658:i32)
        n322 = Greater Or Equal To 0?(x=w658) -> (x >= 0?=w657:bool)
        n323 = property on="多列列表框" class="MCListbox (严格)"() -> (error out=w662:errorcluster, "TopLeft"=w663:T16)  [unwired: 2 in, 1 out]
        n324 = Select(t=w658, s=w657, f=0) -> (s? t:f=w659:i32)
        n325 = Bundle By Name(cluster=w663, "Row"=w659) -> (w664:T16)
        n326 = property on="多列列表框" class="MCListbox (严格)"(error in=w662, "TopLeft"=w664) -> ()  [unwired: 1 in, 2 out]
      }
    }
    n327 = while {
      tunnel: w458 -> [w640]
      shift-right: [w636] -> _
      shift-left: _ -> [w637]
      shift-right: [w626] -> _
      shift-left: _ -> [w638]
      shift-right: [w628] -> _
      shift-left: _ -> [w635]
      tunnel: w459 -> [w627]
      shift-right: [w633] -> _
      shift-left: _ -> [w632]
      tunnel: w454 -> [w633]
      stop <- TRUE stop-if-true
      n328 = Not Equal?(x=w632, y=w633) -> (x != y?=w631:bool)
      n329 = global read "总磷总氮断电保存全局变量.vi" "流程路径"() -> (w628:path)
      n330 = Not Equal To 0?(x=w627) -> (x != 0?=w629:bool)
      n331 = Not Equal?(x=w635, y=w628) -> (x != y?=w630:bool)
      n332 = Compound Arithmetic op=OR ("复合运算")(w629, w630, w631) -> (w634:bool)
      n333 = case shown="真" w634 {
        tunnel: [w642 w652] -> w626
        tunnel: [w641 w651] -> w636
        tunnel: w640 -> [_ w646]
        tunnel: w638 -> [w642 _]
        tunnel: w637 -> [w641 _]
        tunnel: w628 -> [_ w645]
        tunnel: w627 -> [_ w644]
        frame False {
        }
        frame True {
          n334 = call "斯坦道XML解析.vi"("工作状态"=w644, "添加的路径"=w645, "参数簇"=w646) -> ("简易步骤名称"=→"简易步骤名称":string, "步骤时间"=w647:string[], "步骤名"=w649:string[])  [unwired: 6 in]
          n335 = for {
            tunnel: w649 -> [_] mode=indexing
            tunnel: [w653] -> w650 mode=indexing
            i -> [w653]
          }
          n336 = Build Array(w649, w647) -> (w648:string[][])
          n337 = Transpose 2D Array(2D array=w648) -> (transposed array=w651:string[][])
          n338 = Number To Decimal String(number=w650) -> (decimal integer string=w652:string[])  [unwired: 1 in]
        }
      }
      n339 = property on="多列列表框" class="MCListbox (严格)"("ItemNames"=w636, "RowHdrs[]"=w626) -> ()  [unwired: 2 in, 2 out]
      n340 = Array Size(array=w626) -> (size(s)=→"总步数":i32)
    }
    n341 = Multiply(x=w451, y=100.0) -> (x*y=w448:dbl)
    "滑动杆" <- w448
    n342 = case shown="真" w472 {
      tunnel: w470 -> [_ w529]
      tunnel: w471 -> [_ w526]
      tunnel: w449 -> [_ w524]
      frame False {
      }
      frame True {
        n343 = case shown="2" w529 {
          selector: w529 -> [w536 _ _ _ _ _ _ _ _ _ _ _]
          tunnel: [w535 "【水样测试】" ("字符串") w539 "【零点核查】" ("字符串") "【跨度核查】" ("字符串") "【空白测试】" ("字符串") "【平行样测试】" ("字符串") "【加标回收】" ("字符串") "【空白校准】" ("字符串") "【标样校准】" ("字符串") "【单步调试】" ("字符串") "【简易流程】" ("字符串")] -> w534
          tunnel: w524 -> [_ _ w538 _ _ _ _ _ _ _ _ _]
          frame 0, Default {
            n344 = Number To Decimal String(number=w536) -> (decimal integer string=w535:string)  [unwired: 1 in]
          }
          frame 1 {
          }
          frame 2 {
            n345 = case shown="5" w538 {
              tunnel: ["【标样核查】" ("字符串") "【快捷测试】" ("字符串")] -> w539
              frame 0, Default {
              }
              frame 5 {
              }
            }
          }
          frame 3 {
          }
          frame 4 {
          }
          frame 5 {
          }
          frame 6 {
          }
          frame 7 {
          }
          frame 8 {
          }
          frame 9 {
          }
          frame 254 {
          }
          frame 255 {
          }
        }
        n346 = call "id参数转换.vi"("id"=w526) -> ("table输出"=w525:string)  [unwired: 9 in, 1 out]
        n347 = Concatenate Strings("<<" ("字符串"), w534, "启动" ("字符串")) -> (w533:string)
        n348 = Get Date/Time In Seconds() -> (seconds since 1Jan1904=w531:timestamp)
        n349 = Bundle By Name(cluster=T15 {"时间标识"=timestamp(0 s since 1904-01-01), "设备"="", "日志信息"="", "流程参数"=""} ("data in"), "时间标识"=w531, "设备"=w525, "日志信息"=w533) -> (w530:T15)
        n350 = call "总磷总氮操作日志.vi"("data in"=w530) -> ()  [unwired: 10 in, 1 out]
      }
    }
    n351 = case shown="真" w467 {
      tunnel: w470 -> [_ w489]
      tunnel: w471 -> [_ w502]
      tunnel: w449 -> [_ w487]
      frame False {
      }
      frame True {
        n352 = case shown="2" w489 {
          selector: w489 -> [w509 _ _ _ _ _ _ _ _ _ _ _]
          tunnel: [w508 "【水样测试】" ("字符串") w512 "【零点核查】" ("字符串") "【跨度核查】" ("字符串") "【空白测试】" ("字符串") "【平行样测试】" ("字符串") "【加标回收】" ("字符串") "【空白校准】" ("字符串") "【标样校准】" ("字符串") "【单步调试】" ("字符串") "【简易流程】" ("字符串")] -> w490
          tunnel: w487 -> [_ _ w511 _ _ _ _ _ _ _ _ _]
          frame 0, Default {
            n353 = Number To Decimal String(number=w509) -> (decimal integer string=w508:string)  [unwired: 1 in]
          }
          frame 1 {
          }
          frame 2 {
            n354 = case shown="5" w511 {
              tunnel: ["【标样核查】" ("字符串") "【快捷测试】" ("字符串")] -> w512
              frame 0, Default {
              }
              frame 5 {
              }
            }
          }
          frame 3 {
          }
          frame 4 {
          }
          frame 5 {
          }
          frame 6 {
          }
          frame 7 {
          }
          frame 8 {
          }
          frame 9 {
          }
          frame 254 {
          }
          frame 255 {
          }
        }
        n355 = global read "VAR总磷总氮全局变量.vi" "状态告警区"() -> (w500:T7)
        n356 = call "id参数转换.vi"("id"=w502) -> ("table输出"=w501:string)  [unwired: 9 in, 1 out]
        n357 = Unbundle By Name(w500) -> ("F0"=w499:sgl, "F1"=w498:sgl, "F2"=w497:sgl, "F3"=w496:sgl, "id"=w495:u16, "flowid"=w494:u16, "量程"=w493:u16)
        n358 = Format Into String(format string="F0=%#f,F1=%#f,F2=%#f,F3=%#f,Flow=%d-%-d-%-d" ("格式字符串"), w499, w498, w497, w496, w495, w494, w493) -> (resulting string=w491:string)  [unwired: 2 in, 1 out]
        n359 = Concatenate Strings(w490, "停止" ("字符串"), ">>" ("字符串")) -> (w507:string)
        n360 = Get Date/Time In Seconds() -> (seconds since 1Jan1904=w505:timestamp)
        n361 = Bundle By Name(cluster=T15 {"时间标识"=timestamp(0 s since 1904-01-01), "设备"="", "日志信息"="", "流程参数"=""} ("data in"), "时间标识"=w505, "设备"=w501, "日志信息"=w507, "流程参数"=w491) -> (w504:T15)
        n362 = call "总磷总氮操作日志.vi"("data in"=w504) -> ()  [unwired: 10 in, 1 out]
      }
    }
    n363 = global write "VAR总磷总氮全局变量.vi" "测试进度"(w448) -> ()
    n364 = Wait (ms)(milliseconds to wait=u32 1000 ("等待时间（毫秒）")) -> ()  [unwired: 1 out]
  }
  n365 = case shown="\"Bad\", 默认" w10 {
    tunnel: w9 -> [w665 w669]
    tunnel: [w665 w666] -> w8
    frame "Bad", Default {
    }
    frame "Idle" {
      n366 = invoke class="VI" method="Run VI"(reference=w669, "Wait until done"=FALSE ("结束前等待"), "Auto Dispose Ref"=TRUE ("自动销毁引用")) -> (reference out=w666:refnum<vi>)  [unwired: 2 in, 4 out]
    }
  }
  n367 = case shown="\"Bad\", 默认" w14 {
    tunnel: w13 -> [w670 w674]
    tunnel: [w670 w671] -> w12
    frame "Bad", Default {
    }
    frame "Idle" {
      n368 = invoke class="VI" method="Run VI"(reference=w674, "Wait until done"=FALSE ("结束前等待"), "Auto Dispose Ref"=TRUE ("自动销毁引用")) -> (reference out=w671:refnum<vi>)  [unwired: 2 in, 4 out]
    }
  }
  n369 = while {
    tunnel: w21 -> [w678]
    tunnel: w19 -> [w677]
    tunnel: w12 -> [w676]
    tunnel: w8 -> [w675]
    stop <- FALSE stop-if-true
    n370 = event shown="[7] \"停止\": 值改变" {
      selector: _ -> [_ _ _ _ _ _ _ _ _ _ _ _ _]
      dyn-events: _ -> [_ _ _ _ _ _ _ _ _ _ _ _ _]
      timeout: _ -> [_ _ _ _ _ _ _ _ _ _ _ _ _]
      tunnel: w678 -> [_ _ _ _ _ w690 _ w699 _ _ _ _ _]
      tunnel: w677 -> [_ _ _ _ _ _ _ w698 _ _ _ _ _]
      tunnel: w676 -> [_ _ _ _ _ _ _ _ w706 _ _ _ _]
      tunnel: w675 -> [_ _ _ _ _ _ _ _ _ _ _ w712 _]
      event Timeout {
        n371 = event-data() -> ()  [unwired: 1 in, 3 out]
      }
      event "温度曲线": Value Change {
        n372 = event-data() -> ()  [unwired: 1 in, 6 out]
        n373 = call "温度曲线显示.vi"() -> ()  [unwired: 12 in]
      }
      event "启动参数设置": Value Change {
        n374 = event-data() -> ()  [unwired: 1 in, 6 out]
        n375 = call "启动参数设置.vi"() -> ()  [unwired: 12 in]
      }
      event "布尔": Value Change {
        n376 = event-data() -> ("NewVal"=w680:bool)  [unwired: 1 in, 5 out]
        n377 = case shown="假" w680 {
          frame False {
            n378 = global write "VAR总磷总氮全局变量.vi" "权限等级"(enum16{"一级权限", "二级权限", "三级权限", "超级权限"}."一级权限" ("权限等级")) -> ()
          }
          frame True {
            n379 = global read "VAR总磷总氮全局变量.vi" "权限密码"() -> (w684:u32[])
            n380 = global read "VAR总磷总氮全局变量.vi" "权限等级"() -> (w682:enum16{"一级权限", "二级权限", "三级权限", "超级权限"})
            n381 = call "密码权限设置.vi"("权限输入"=w682, "权限密码"=w684) -> ("权限输出"=w683:enum16{"一级权限", "二级权限", "三级权限", "超级权限"})  [unwired: 9 in]
            n382 = global write "VAR总磷总氮全局变量.vi" "权限等级"(w683) -> ()
          }
        }
      }
      event "权限等级": Mouse Down {
        n383 = event-data() -> ()  [unwired: 1 in, 8 out]
        n384 = global read "VAR总磷总氮全局变量.vi" "权限密码"() -> (w687:u32[])
        n385 = global read "VAR总磷总氮全局变量.vi" "权限等级"() -> (w685:enum16{"一级权限", "二级权限", "三级权限", "超级权限"})
        n386 = call "密码权限设置.vi"("权限输入"=w685, "权限密码"=w687) -> ("权限输出"=w686:enum16{"一级权限", "二级权限", "三级权限", "超级权限"})  [unwired: 9 in]
        n387 = global write "VAR总磷总氮全局变量.vi" "权限等级"(w686) -> ()
      }
      event "手动启动": Value Change {
        n388 = event-data() -> ()  [unwired: 1 in, 6 out]
        n389 = call "总磷总氮启动参数对话框.vi"() -> ("确认"=w688:bool, "元素"=w689:cluster{"命令":string, "data":variant})  [unwired: 10 in]
        n390 = case shown="真" w688 {
          tunnel: w690 -> [_ w693]
          tunnel: w689 -> [_ w692]
          frame False {
          }
          frame True {
            n391 = Flush Queue(queue=w693) -> (queue out=w691:refnum<queue>)  [unwired: 1 in, 2 out]
            n392 = Enqueue Element(queue=w691, element=w692) -> ()  [unwired: 2 in, 3 out]
          }
        }
      }
      event "调试": Value Change {
        n393 = event-data() -> ()  [unwired: 1 in, 6 out]
        n394 = call "总磷单步调试对话框.vi"() -> ()  [unwired: 12 in]
      }
      event "停止": Value Change {
        n395 = event-data() -> ()  [unwired: 1 in, 6 out]
        n396 = global read "VAR总磷总氮全局变量.vi" "状态告警区"() -> (w696:T7)
        n397 = Send Notification(notification=TRUE ("通知"), notifier=w698) -> ()  [unwired: 1 in, 2 out]
        n398 = Unbundle By Name(w696) -> ("id"=w695:u16)
        n399 = case shown="3, 92" w695 {
          tunnel: [_ cluster{"命令":string, "data":variant} {"命令"="启动", "data"=variant(cluster{"站号":u16, "控制命令输出":u16[]} {"站号"=1, "控制命令输出"=[2816]})} ("元素") cluster{"命令":string, "data":variant} {"命令"="启动", "data"=variant(cluster{"站号":u16, "控制命令输出":u16[]} {"站号"=2, "控制命令输出"=[2816]})} ("元素") cluster{"命令":string, "data":variant} {"命令"="启动", "data"=variant(cluster{"站号":u16, "控制命令":u16[]} {"站号"=3, "控制命令"=[2816]})} ("元素")] -> w694
          frame 0, Default {
          }
          frame 1, 131 {
          }
          frame 2, 76 {
          }
          frame 3, 92 {
          }
        }
        n400 = Enqueue Element(queue=w699, element=w694) -> ()  [unwired: 2 in, 3 out]
      }
      event "参数设置", "参数查询": Value Change {
        n401 = event-data() -> ()  [unwired: 1 in, 6 out]
        n402 = invoke on="子面板" class="SubPnl" method="Remove VI"() -> (error out=w707:errorcluster)  [unwired: 3 in, 2 out]
        n403 = property on="参数查询" class="Bool"("Visible"=FALSE ("可见")) -> ()  [unwired: 2 in, 2 out]
        n404 = property on="仪器校准" class="Bool"("Visible"=TRUE ("可见")) -> ()  [unwired: 2 in, 2 out]
        n405 = global write "VAR总磷总氮全局变量.vi" "页面"(enum16{"主页", "参数页", "校准页"}."参数页" ("页面")) -> ()
        n406 = property on="窗格" class="Pane"("Origin"=T6 {"Horizontal"=0, "Vertical"=640} ("原点")) -> ()  [unwired: 2 in, 2 out]
        n407 = invoke on="子面板" class="SubPnl" method="Insert VI"(error in=w707, "VI Ref"=w706) -> ()  [unwired: 2 in, 4 out]
      }
      event "修改系列号": Value Change {
        n408 = event-data() -> ()  [unwired: 1 in, 6 out]
        n409 = call "写入系列号对话框.vi"() -> ()  [unwired: 12 in]
      }
      event "流程写入": Value Change {
        n410 = event-data() -> ()  [unwired: 1 in, 6 out]
        n411 = call "流程复合写入.vi"() -> ()  [unwired: 12 in]
      }
      event "仪器校准": Value Change {
        n412 = event-data() -> ()  [unwired: 1 in, 6 out]
        n413 = invoke on="子面板" class="SubPnl" method="Remove VI"() -> (error out=w713:errorcluster)  [unwired: 3 in, 2 out]
        n414 = property on="参数查询" class="Bool"("Visible"=TRUE ("可见")) -> ()  [unwired: 2 in, 2 out]
        n415 = property on="仪器校准" class="Bool"("Visible"=FALSE ("可见")) -> ()  [unwired: 2 in, 2 out]
        n416 = global write "VAR总磷总氮全局变量.vi" "页面"(enum16{"主页", "参数页", "校准页"}."校准页" ("页面")) -> ()
        n417 = invoke on="子面板" class="SubPnl" method="Insert VI"(error in=w713, "VI Ref"=w712) -> ()  [unwired: 2 in, 4 out]
      }
      event "返回": Value Change {
        n418 = event-data() -> ()  [unwired: 1 in, 6 out]
        n419 = global write "VAR总磷总氮全局变量.vi" "页面"(enum16{"主页", "参数页", "校准页"}."主页" ("页面")) -> ()
        n420 = property on="窗格" class="Pane"("Origin"=T6 {"Horizontal"=0, "Vertical"=0} ("原点")) -> ()  [unwired: 2 in, 2 out]
      }
    }
  }
